vi "_WriteTagTemplate.vi"(8 "error in (no error)":errorcluster, 9 "Value":variant, 10 "name":string, 11 "TagMap":refnum<data-value>) -> (0 "error out":errorcluster, 3 "TagMap(dup)":refnum<data-value>)   [LabVIEW 2017, in "WriteTag.xnode"]
uses:
  WriteTag.xnode
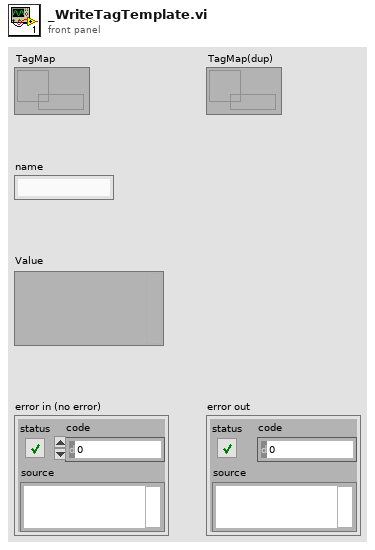
[diagram p1: front panel]
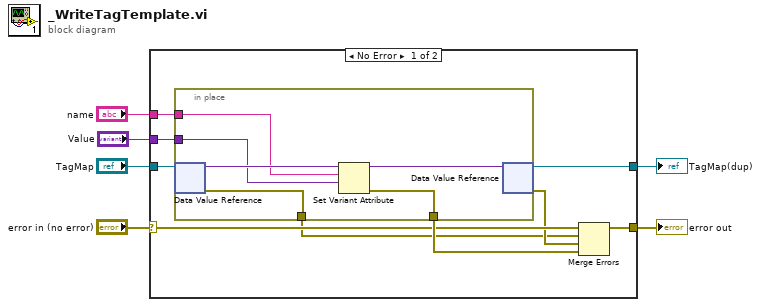
[diagram p0: block diagram]
diagram:
  n1 = case shown="No Error" "error in (no error)" {
    selector: "error in (no error)" -> [w13 w23]
    tunnel: [w14 w23] -> w6
    tunnel: "name" -> [w10 _]
    tunnel: [w9 w22] -> w3
    tunnel: "TagMap" -> [w8 w22]
    tunnel: "Value" -> [w7 _]
    frame No Error {
      n2 = in-place "In Place Element Structure" {
        in-place-border: w10 -> [w19]
        in-place-border: [w17] -> w11
        in-place-border: [w18] -> w15
        in-place-border: w7 -> [w16]
        n3 = in-place-dvr #1(w8) -> (w21:variant, w17:errorcluster)
        n4 = Set Variant Attribute(Variant=w21, name=w19, value=w16) -> (Variant out=w20:variant, error out=w18:errorcluster)  [unwired: 1 in, 1 out]
        n5 = in-place-dvr #1(w20) -> (w9:refnum<data-value>, w12:errorcluster)
      }
      n6 = Merge Errors(w13, w11, w12, w15) -> (w14:errorcluster)
    }
    frame Error {
    }
  }
  "error out" <- w6
  "TagMap(dup)" <- w3
